vi "CamCalibrationTest.vi"() -> ()   [LabVIEW 2019]
panel:
  out "ImgOut":T1(plugin-control)
  out "CalImgOut":T1(plugin-control)
  in  "Stop Button":bool
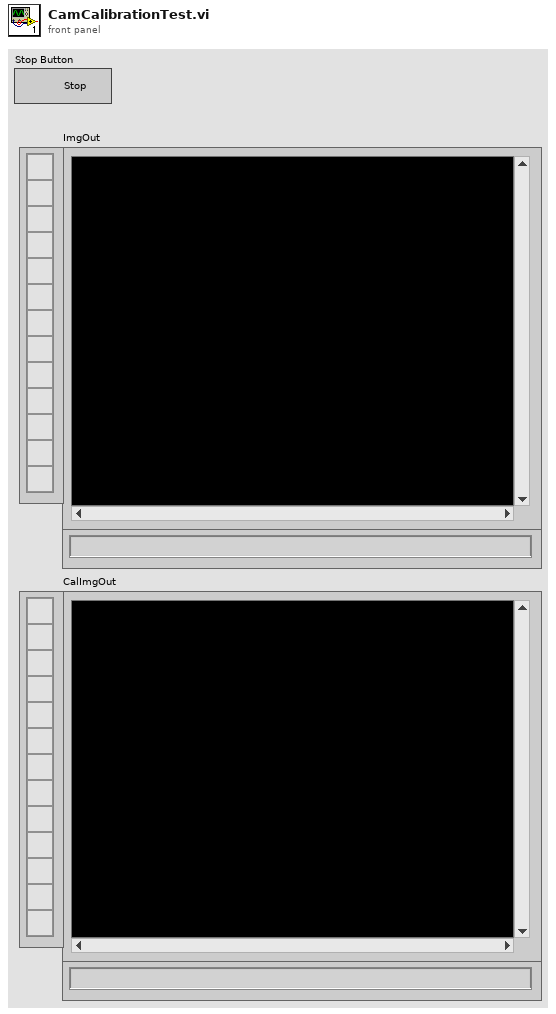
[diagram p1: front panel]
types:
  T1 = typedef "IMAQ Image.ctl" = refnum<image>
  T2 = typedef "Image Type" = u32
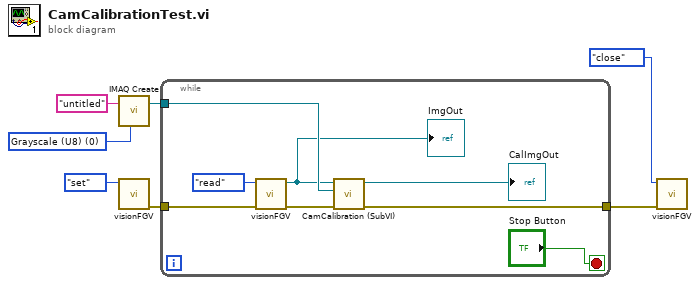
[diagram p0: block diagram]
diagram:
  w1 = T2 0 items=["Grayscale (U8)", "Grayscale (I16)", "Grayscale (SGL)", "Complex (CSG)", "RGB (U32)", "HSL (U32)", "RGB (U64)", "Grayscale (U16)"] ("Image Type")
  n1 = call "IMAQ Create"("Image Name"="untitled", "Image Type"=w1) -> ("New Image"=w3:T1)  [unwired: 3 in, 1 out]
  n2 = call "visionFGV.vi"("Function"=enum16{"set", "read", "close"}."set") -> ("error out"=w6:errorcluster)  [unwired: 9 in, 1 out]
  n3 = while {
    tunnel: w6 -> [w10]
    tunnel: [w13] -> w4
    tunnel: w3 -> [w11]
    stop <- "Stop Button" stop-if-true
    n4 = call "visionFGV.vi"("Error In"=w10, "Function"=enum16{"set", "read", "close"}."read") -> ("error out"=w9:errorcluster, "Image Out fgv"=w8:T1)  [unwired: 8 in]
    "ImgOut" <- w8
    n5 = call "CamCalibration (SubVI).vi"("error in"=w9, "Image Dst"=w11, "Image In"=w8) -> ("error out"=w13:errorcluster, "Image Out"=→"CalImgOut":T1)  [unwired: 7 in]
  }
  n6 = call "visionFGV.vi"("Error In"=w4, "Function"=enum16{"set", "read", "close"}."close") -> ()  [unwired: 8 in, 2 out]
